vi "Pressure_control_subVI.vi"(1 "User-defined\nsequence":string[][](array[string]), 5 "references in":T4, 9 "pressure controlk / turbo / current step / present sec/run seq/press settings":T2, 12 "DAQ IDs in":T5) -> (3 "pressure":cluster{"pressure":dbl}, 4 "press/RH/gas/vapor":T6, 6 "pressure params out":T3, 8 "seq on/end time/current step":T1, 14 "date/time string":string, 15 "DAQ IDs out":T7)   [LabVIEW 2014]
uses:
  <vilib>/DAQmx/read.llb/DAQmx Read (Analog 1D DBL NChan 1Samp).vi
  <vilib>/DAQmx/write.llb/DAQmx Write (Analog 1D DBL NChan 1Samp).vi
  <vilib>/DAQmx/write.llb/DAQmx Write (Digital Bool 1Line 1Point).vi
panel:
  out "sequence end time":timestamp
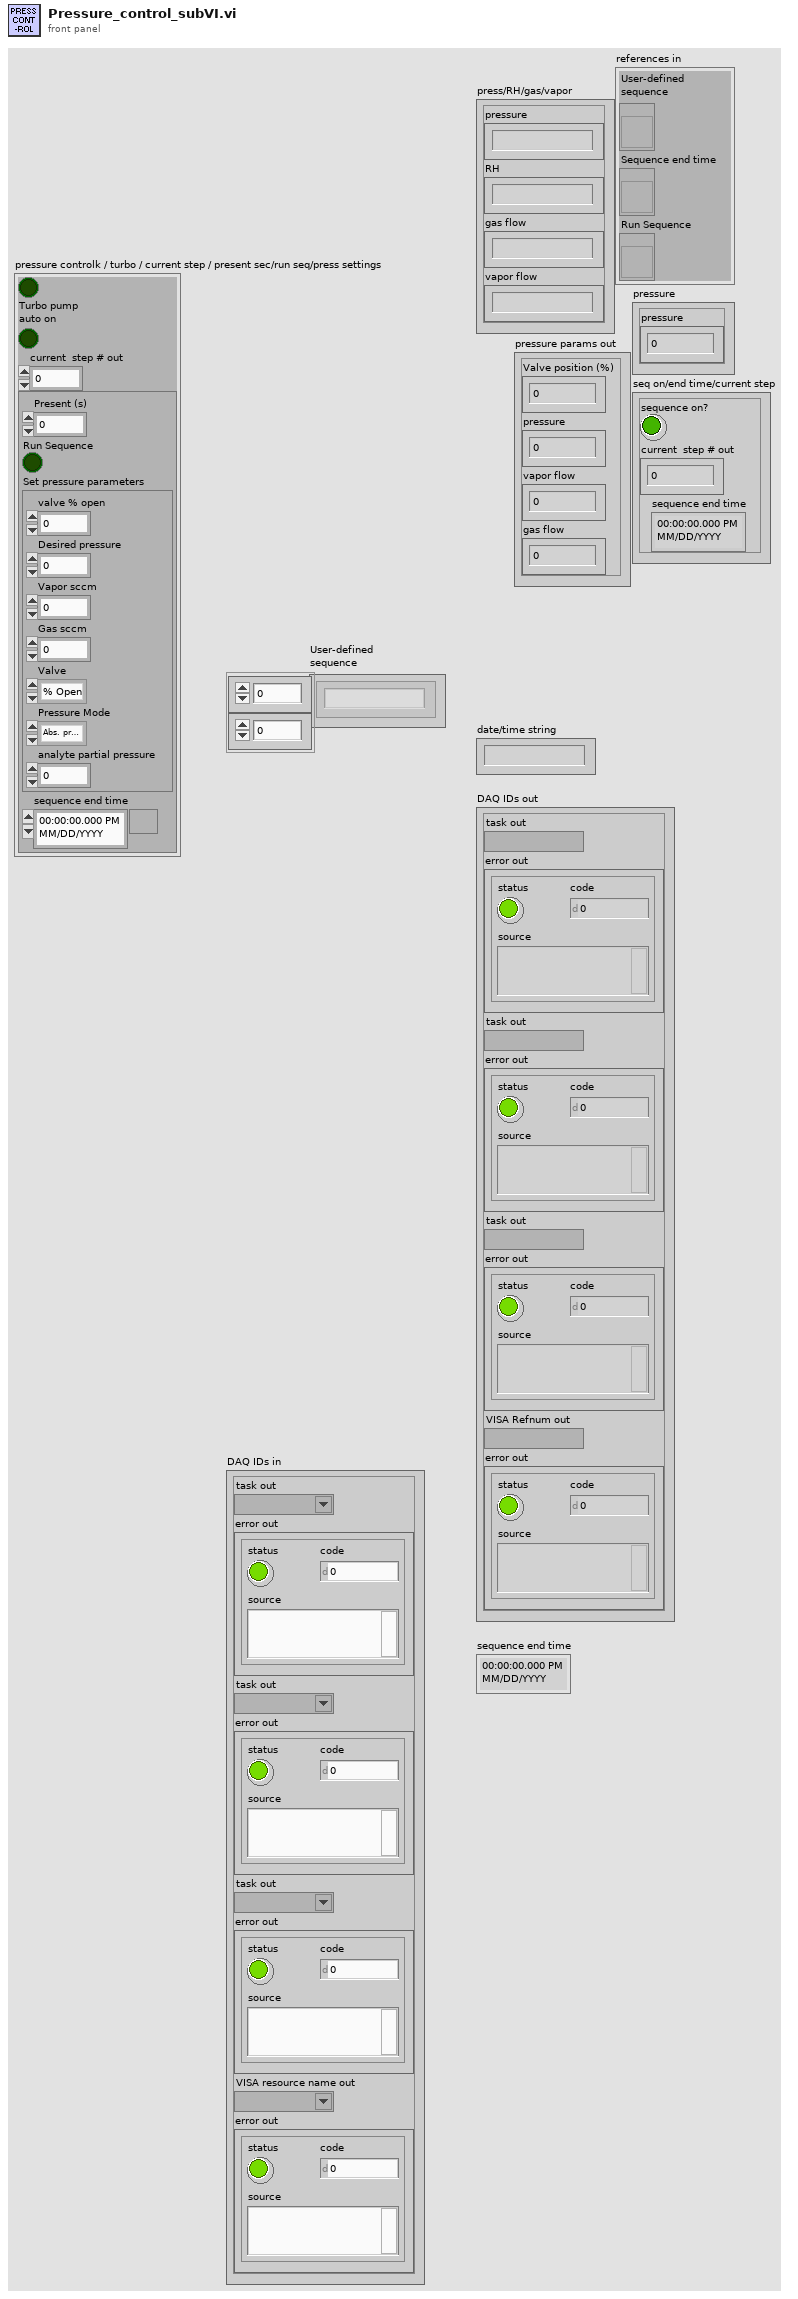
[diagram p1: front panel]
types:
  T1 = cluster{"sequence on?":bool, "current  step # out":i32, "sequence end time":timestamp}
  T2 = cluster{bool, "Turbo pump\nauto on":bool, "current  step # out":i32, cluster{"Present (s)":dbl, "Run Sequence":bool, "Set pressure parameters":cluster{"valve % open":dbl, "Desired pressure":dbl, "Vapor sccm":sgl, "Gas sccm":sgl, "Valve":enum32{"% Open", "Torr "}, "Pressure Mode":enum32{"Abs. pressure", " Part. pressure"}, "analyte partial pressure":dbl}, "sequence end time":timestamp}}
  T3 = cluster{"Valve position (%)":dbl, "pressure":dbl, "vapor flow":dbl, "gas flow":dbl}
  T4 = cluster{"User-defined\nsequence":refnum<vi>, "Sequence end time":refnum<vi>, "Run Sequence":refnum<vi>}
  T5 = cluster{"task out":refnum<k21>, "error out":errorcluster, "task out":refnum<k21>, "error out":errorcluster, "task out":refnum<k21>, "error out":errorcluster, "VISA resource name out":refnum<visa-resource-name>, "error out":errorcluster}
  T6 = cluster{"pressure":string, "RH":string, "gas flow":string, "vapor flow":string}
  T7 = cluster{"task out":refnum<k21>, "error out":errorcluster, "task out":refnum<k21>, "error out":errorcluster, "task out":refnum<k21>, "error out":errorcluster, "VISA Refnum out":refnum<visa-resource-name>, "error out":errorcluster}
  T8 = cluster{"Present (s)":dbl, "Run Sequence":bool, "Set pressure parameters":cluster{"valve % open":dbl, "Desired pressure":dbl, "Vapor sccm":sgl, "Gas sccm":sgl, "Valve":enum32{"% Open", "Torr "}, "Pressure Mode":enum32{"Abs. pressure", " Part. pressure"}, "analyte partial pressure":dbl}, "sequence end time":timestamp}
  T9 = enum8{"Enabled", "Disabled", "Disabled and Grayed Out"}
  T10 = cluster{"valve % open 2":dbl, "Pressure Control":u32, "Desired pressure":dbl, "Disabled":enum8{"Enabled", "Disabled", "Disabled and Grayed Out"}}
  T11 = cluster{"valve % open 2":dbl, "Pressure Control":u32, "Desired pressure":dbl}
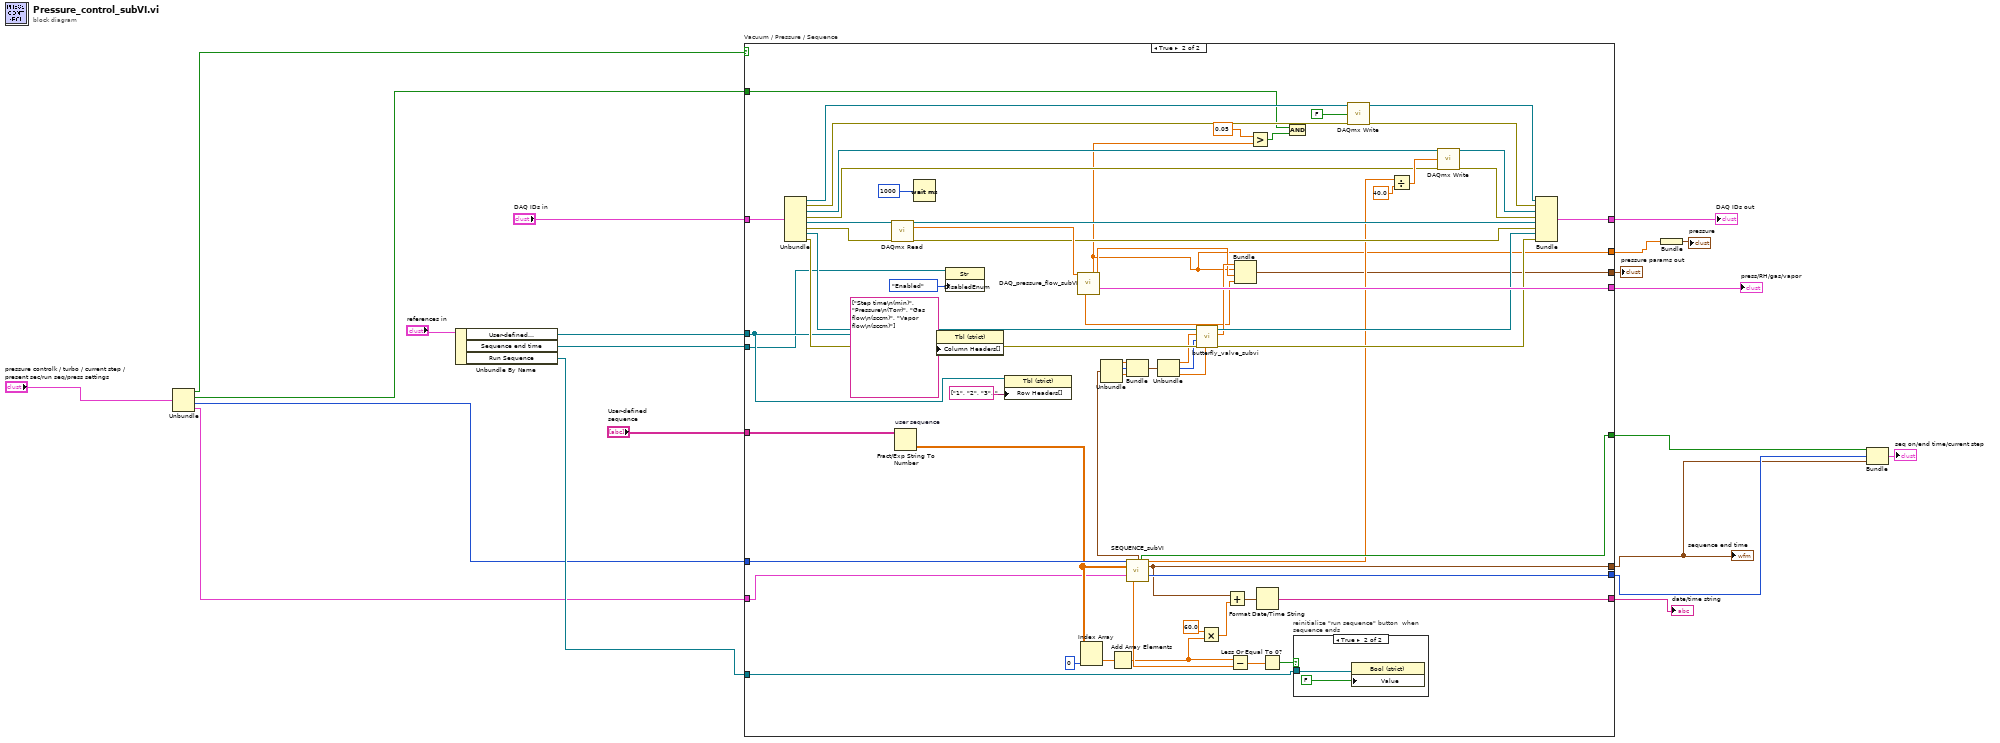
[diagram p0: block diagram]
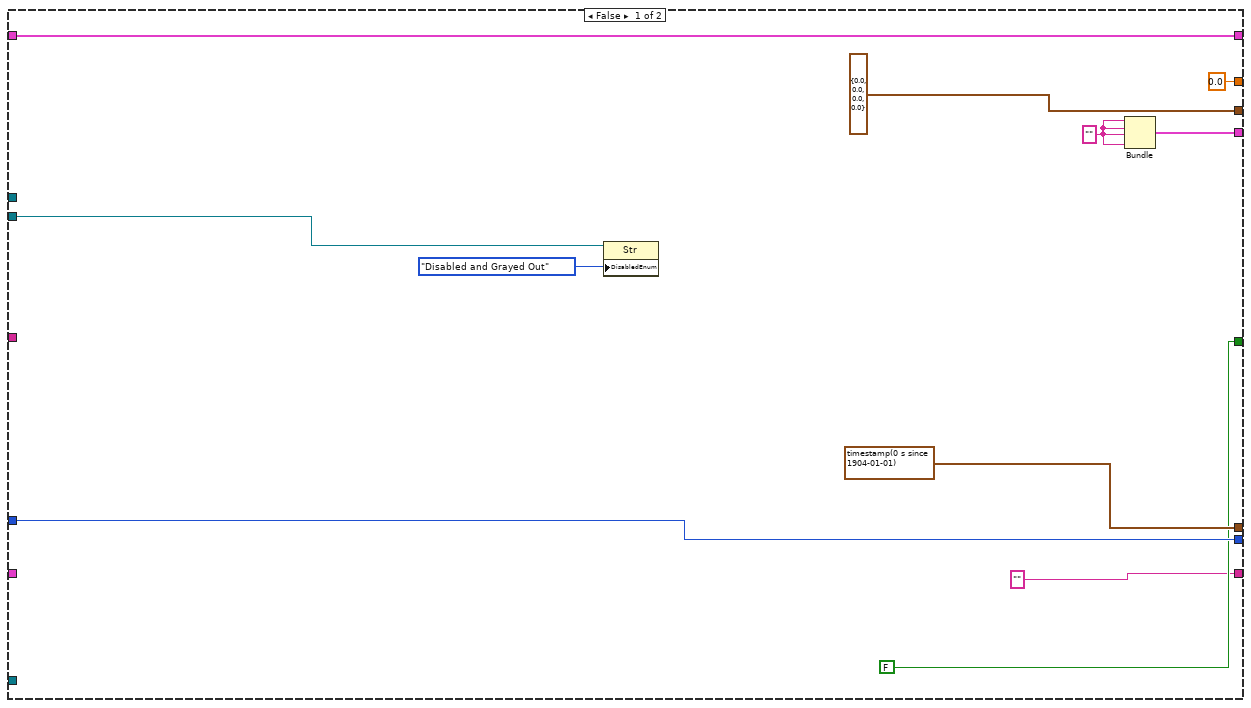
[diagram p2: hidden frame]
diagram:
  n1 = Unbundle("pressure controlk / turbo / current step / present sec/run seq/press settings") -> (w6:bool, "Turbo pump\nauto on"=w5:bool, "current  step # out"=w4:i32, w7:T8)
  n2 = Unbundle By Name("references in") -> ("User-defined\nsequence"=w16:refnum<vi>, "Sequence end time"=w15:refnum<vi>, "Run Sequence"=w14:refnum<vi>)
  n3 = case "Vacuum / Pressure / Sequence" shown="True" w6 {
    tunnel: "DAQ IDs in" -> [w26 w92]
    tunnel: w4 -> [w32 w79]
    tunnel: [w32 w82] -> w3
    tunnel: [FALSE w74] -> w13
    tunnel: [timestamp(0 s since 1904-01-01) ("seconds since 1Jan1904") w73] -> w2
    tunnel: w7 -> [_ w34]
    tunnel: [w28 w55] -> w19
    tunnel: [w26 w46] -> w20
    tunnel: w5 -> [_ w41]
    tunnel: "User-defined\nsequence" -> [_ w40]
    tunnel: ["" ("date/time string") w39] -> w12
    tunnel: [T3 {"Valve position (%)"=0.0, "pressure"=0.0, "vapor flow"=0.0, "gas flow"=0.0} w38] -> w11
    tunnel: w15 -> [w23 w35]
    tunnel: w14 -> [_ w37]
    tunnel: w16 -> [_ w36]
    tunnel: [0.0 ("pressure") w33] -> w10
    frame False {
      w27 = ""
      n4 = property on="Property Node" class="Str"(reference=w23, "DisabledEnum"=T9."Disabled and Grayed Out" ("Disabled")) -> ()  [unwired: 1 in, 2 out]
      n5 = Bundle(w27, w27, w27, w27) -> (w28:cluster{string, string, string, string})  [unwired: 1 in]
    }
    frame True {
      n6 = Unbundle(w92) -> ("task out"=w85:refnum<k21>, "error out"=w84:errorcluster, "task out"=w86:refnum<k21>, "error out"=w87:errorcluster, "task out"=w88:refnum<k21>, "error out"=w89:errorcluster, "VISA resource name out"=w90:refnum<visa-resource-name>, "error out"=w91:errorcluster)
      n7 = call-poly <vilib>:"DAQmx Read.vi"("task/channels in"=w88, "error in"=w89) -> ("task out"=w50:refnum<k21>, "data"=w95:dbl[], "error out"=w49:errorcluster)  [unwired: 11 in]
      n8 = Fract/Exp String To Number "user sequence"(string=w40) -> (number=w66:dbl[][])  [unwired: 3 in, 1 out]
      n9 = Wait (ms)(milliseconds to wait=u32 1000) -> ()  [unwired: 1 out]
      n10 = property on="Property Node" class="Tbl (strict)"(reference=w36, "Column Headers[]"=string[] ["Step time\n(min)", "Pressure\n(Torr)", "Gas flow\n(sccm)", "Vapor flow\n(sccm)"] ("Column Header Strings[]")) -> ()  [unwired: 1 in, 2 out]
      n11 = property on="Property Node" class="Str"(reference=w35, "DisabledEnum"=T9."Enabled" ("Disabled")) -> ()  [unwired: 1 in, 2 out]
      n12 = property on="Property Node" class="Tbl (strict)"(reference=w36, "Row Headers[]"=string[] ["1", "2", "3", "4", "5", "6", "7", "8", "9", "10", "11", "12", "13", "14", "15", "16", "17", "18", "19", "20", "21", "22", "23", "24", "25", "26", "27", "28", "29", "30", "31", "32", "33", "34", "35", "36", "37", "38", "39", "40"] ("Row Header Strings[]")) -> ()  [unwired: 1 in, 2 out]
      n13 = call "DAQ_pressure_flow_subVI.vi"("vac press"=w95) -> ("pressure"=w33:dbl, "vapor flow"=w44:dbl, "press/RH/gas/vapor"=w55:T6, "gas flow"=w43:dbl)  [unwired: 10 in, 1 out]
      n14 = Index Array(array=w66, index (col)=0 ("disabled index (col)")) -> (element=w81:dbl[])  [unwired: 1 in]
      n15 = Add Array Elements(numeric array=w81) -> (sum=w68:dbl)
      n16 = call "SEQUENCE_subVI.vi"("current step # in"=w79, "user sequence in"=w66, "input data"=w34) -> ("pressure control settings out"=w64:T10, "sequence on?"=w74:bool, "vapor and gas flow out"=w42:dbl[], "sequence end time"=w73:timestamp, "current  step # out"=w82:i32, "time spent running"=w78:dbl)  [unwired: 7 in]
      n17 = Unbundle(w64) -> ("valve % open 2"=w63:dbl, "Pressure Control"=w62:u32, "Desired pressure"=w58:dbl)  [unwired: 1 out]
      n18 = Bundle("valve % open 2"=w63, "Pressure Control"=w62, "Desired pressure"=w58) -> (w61:T11)  [unwired: 1 in]
      n19 = Unbundle(w61) -> ("valve % open 2"=w60:dbl, "Pressure Control"=w59:u32, "Desired pressure"=w57:dbl)
      n20 = call "butterfly_valve_subvi.vi"("Desired pressure"=w57, "error in (no error)"=w91, "Pressure Control"=w59, 10:w60, "VISA Refnum in"=w90) -> ("error out"=w47:errorcluster, "Valve position (%)"=w45:dbl, "VISA Refnum out"=w48:refnum<visa-resource-name>)  [unwired: 4 in]
      n21 = Multiply(x=60.0 ("y"), y=w68) -> (x*y=w71:dbl)
      n22 = Add(x=w73, y=w71) -> (x+y=w70:timestamp)
      n23 = Subtract(x=w68, y=w78) -> (x-y=w75:dbl)
      n24 = Bundle("Valve position (%)"=w45, "pressure"=w33, "vapor flow"=w44, "gas flow"=w43) -> (w38:T3)  [unwired: 1 in]
      n25 = Greater?(x=0.05, y=w33) -> (0:w56:bool)
      n26 = Format Date/Time String(seconds (now)=w70) -> (date/time string=w39:string)  [unwired: 2 in]
      n27 = Less Or Equal To 0?(x=w75) -> (x <= 0?=w65:bool)
      n28 = And(x=w41, y=w56) -> ()  [unwired: 1 out]
      n29 = case "reinitialize \"run sequence\" button  when sequence ends" shown="True" w65 {
        tunnel: w37 -> [_ w97]
        frame False {
        }
        frame True {
          n30 = property on="Property Node" class="Bool (strict)"(reference=w97, "Value"=FALSE ("Run Sequence")) -> ()  [unwired: 1 in, 2 out]
        }
      }
      n31 = call-poly <vilib>:"DAQmx Write.vi"("task/channels in"=w85, "data"=FALSE, "error in"=w84) -> ("task out"=w54:refnum<k21>, "error out"=w53:errorcluster)  [unwired: 10 in, 1 out]
      n32 = Divide(x=w42, y=40.0 ("Waveform")) -> (x/y=w94:dbl[])
      n33 = call-poly <vilib>:"DAQmx Write.vi"("task/channels in"=w86, "data"=w94, "error in"=w87) -> ("task out"=w52:refnum<k21>, "error out"=w51:errorcluster)  [unwired: 10 in, 1 out]
      n34 = Bundle("task out"=w54, "error out"=w53, "task out"=w52, "error out"=w51, "task out"=w50, "error out"=w49, "VISA Refnum out"=w48, "error out"=w47) -> (w46:T7)  [unwired: 1 in]
    }
  }
  "date/time string" <- w12
  "DAQ IDs out" <- w20
  "press/RH/gas/vapor" <- w19
  "sequence end time" <- w2
  "pressure params out" <- w11
  n35 = Bundle("pressure"=w10) -> (→"pressure":cluster{"pressure":dbl})  [unwired: 1 in]
  n36 = Bundle("sequence on?"=w13, "current  step # out"=w3, "sequence end time"=w2) -> (→"seq on/end time/current step":T1)  [unwired: 1 in]
